vi "S4GUI.vi"(7 "Tab ObsEng":enum32{"Obs", "CCD modes", "Eng"}(tab)) -> ()   [LabVIEW 2018]
uses:
  S4GUI/S4GUI.lvclass
  S4GUI/S4GUI.lvclass/S4GUI.ctl
  Interface/Interface.lvclass/Interface.ctl
  Channel/Channel.lvclass/Channel.ctl
  Instrument/Instrument.lvclass/Instrument.ctl
  Device/Optics/Optics.lvclass/Optics.ctl
  Server/Server.lvclass/Server.ctl
  Device/Optics/Opt_Selector/Opt_Selector.lvclass
  C:/Users/devstaff/sparc4/s4gui/Versao ZeroMQ REQ-REP/SPARC4_GUI -20241112/Device/Optics/Optics.lvclass
  Device/Optics/Opt_Continuous/Opt_Continuous.lvclass
  SyncBox/Sync Box.lvclass
  C:/Users/devstaff/sparc4/s4gui/Versao ZeroMQ REQ-REP/SPARC4_GUI -20241112/Server/Server.lvclass
  Acquisition/Acquisition.lvclass
  Instrument/Instrument.lvclass
  Channel/Channel.lvclass
  TelFocus/TelFocus.lvclass
  Interface/Interface.lvclass
  StateMachine/State Machine.lvclass
  TCS/TCS.lvclass
  Publisher/Publisher.lvclass
  Trigger/Trigger.lvclass
  SecMirror/SecMirror.lvclass
  Device/Optics/Optics.lvclass
  Server/Server.lvclass
  Comm/Stream/Stream.lvclass
panel:
  out "GUI version":string
  out "LedExtSync":bool
  out "Name":string
  out "Angle":string
  out "Last Error":string
  in  "Tab Control 3":enum32{"Page 1"}(tab)
  in  "set Observer":bool
  out "Weather":bool
  out "Focus 160":bool
  in  "Observer":string
  out "S4ICSoft":bool
  out "Sync Box":bool
  out "Channel 4":bool
  out "Channel 3":bool
  out "Channel 2":bool
  out "Channel 1":bool
  out "GUIDER":bool
  out "TCSPD":bool
  in  "exit":bool
  out "RA":string
  out "DEC":string
  out "Julian Date":string
  out "Hour Angle":string
  out "Sideral Time":string
  out "Air Mass":string
  out "Date":string
  out "Telescope Focus":string
  out "Outside Temp":string
  out "Wind Speed[Km/h]":string
  out "Pressure":string
  out "Humidity":string
  in  "Project ID":string
  out "error out 8":errorcluster
  out "error out 7":errorcluster
  out "Readout\nRate":u8
  out "error out 6":errorcluster
  out "error out 5":errorcluster
  out "error out 4":errorcluster
  out "error out 3":errorcluster caption="error out"
  out "error out 2":errorcluster caption="error out"
  in  "S4ACS_GUI.lvclass":refnum<class "S4GUI.lvclass">
  out "Panel cooler 4":bool caption="Cooler"
  in  "set keywords":bool
  out "setupCH4":bool caption="Boolean"
  in  "Start ch4":bool
  in  "Pause ch4":bool
  in  "Stop ch4":bool
  in  "Abort ch4":bool
  out "Acq status string ch4":string
  out "setupCH3":bool caption="Boolean"
  in  "Start ch3":bool
  in  "Pause ch3":bool
  in  "Stop ch3":bool
  in  "Abort ch3":bool
  out "Acq status string ch3":string
  out "setupCH1":bool caption="Boolean"
  in  "Pause ch1":bool
  in  "Abort ch1":bool
  in  "Stop ch1":bool
  in  "Start ch1":bool
  out "Acq status string ch1":string
  out "setupCH2":bool caption="Boolean"
  in  "Start ch2":bool
  in  "Pause ch2":bool
  in  "Stop ch2":bool
  in  "Abort ch2":bool
  out "Acq status string ch2":string
  out "RO4":string caption="Read"
  out "G4":string caption="Gain"
  out "B4":string caption="Binn"
  out "PA4":string caption="Pre Amp"
  out "EA4":string caption="Mode"
  out "SI4":string caption="Sub image"
  out "Panel Temp 4":i16 caption="current"
  out "FT4":bool caption="FT"
  out "RO3":string caption="Read"
  out "G3":string caption="Gain"
  out "B3":string caption="Binn"
  out "PA3":string caption="Pre Amp"
  out "EA3":string caption="Mode"
  out "SI3":string caption="Sub image"
  out "Panel cooler 3":bool caption="Cooler"
  out "Panel Temp 3":i16 caption="current"
  out "FT3":bool caption="FT"
  out "RO2":string caption="Read"
  out "G2":string caption="Gain"
  out "B2":string caption="Binn"
  out "PA2":string caption="Pre Amp"
  out "EA2":string caption="Mode"
  out "SI2":string caption="Sub Image"
  out "Panel cooler 2":bool caption="Cooler"
  out "Panel Temp 2":i16 caption="current"
  out "FT2":bool caption="FT"
  out "G1":string caption="Gain"
  out "B1":string caption="Binn"
  out "PA1":string caption="PreAmp"
  out "EA1":string caption="Mode"
  out "SI1":string caption="Sub Image"
  out "FT1":bool caption="FT"
  in  "Tab CH3":enum32{"Acquisition", "CCD temp"}(tab)
  out "Cycles Done ch3":u32(slide) caption="#Cycles Done 1" scale=0.0..1.0
  out "Exposures Done ch3":i32(slide) caption="#Exposures Done 1" scale=0.0..1.0
  in  "#cycles ch3":u32=1 caption="#cycles" min=1 step=1
  in  "Exptime ch3":dbl=1.0 min=1e-05 step=1e-05
  in  "Exp ch3":u32=1 min=1 step=1
  out "Exposure Time ch3":dbl(slide) caption="Exposure Time 0.10" scale=0.0..0.1
  out "Last Image ch3":string caption="Last Image"
  out "Disk Storage ch3":u16(slide) caption="Disk Storage 75%" scale=0.0..100.0
  in  "Ready to OFF 3":bool caption="Ready to Power Off"
  out "Ext Cooling  status 3":bool caption="Ext Cool"
  out "Liquid Type 3":string caption="Liquid Type"
  out "Temp Status 3":string caption="Temp Status"
  out "Curr Temp 3":i16=1 min=1 step=1
  in  "Set Temp 3":bool
  in  "Target Temp 3":i32=1 caption="Target (C)" max=30
  out "Cooler status 3":bool caption="Cooler status"
  in  "Cooler 3":bool caption="Cooler"
  in  "Tab CH1":enum32{"Acquisition", "CCD temp"}(tab)
  out "Exposures Done ch1":i32(slide) caption="#Exposures Done 1" scale=0.0..1.0
  in  "Exptime ch1":dbl=1.0 min=1e-05 step=1e-05 format="%#.6g"
  in  "Exp ch1":u32=1 min=1 step=1
  out "Exposure Time ch1":dbl(slide) caption="Exposure Time 0.10" scale=0.0..0.1
  out "Last Image ch1":string caption="Last Image"
  out "Disk Storage ch1":u16(slide) caption="Disk Storage 52%" scale=0.0..100.0
  out "Cycles Done ch1":u32(slide) caption="#Cycles Done 1" scale=0.0..1.0
  in  "#cycles ch1":u32=1 caption="#cycles" min=1 step=1
  in  "Ready to OFF":bool caption="Ready to Power Off"
  out "Ext Cooling  status 1":bool caption="Ext Cool"
  out "Liquid Type 1":string caption="Liquid Type"
  in  "Set Temp 1":bool
  out "Temp Status 1":string caption="Temp Status"
  out "Cooler status 1":bool caption="Cooler status"
  in  "Target Temp 1":i8=1 caption="Target (C)" max=30
  in  "Cooler 1":bool caption="Cooler"
  out "Curr Temp 1":i16=1 min=1 step=1
  in  "Tab CH4":enum32{"Acquisition", "CCD temp"}(tab)
  out "Cycles Done ch4":u32(slide) caption="#Cycles Done 1" scale=0.0..1.0
  out "Exposures Done ch4":i32(slide) caption="#Exposures Done 1" scale=0.0..1.0
  in  "Exptime ch4":dbl=1.0 min=1e-05 step=1e-05
  in  "Exp ch4":u32=1 min=1 step=1
  in  "#cycles ch4":u32=1 caption="#cycles" min=1 step=1
  out "Exposure Time ch4":dbl(slide) caption="Exposure Time 0.10" scale=0.0..0.1
  out "Last Image ch4":string caption="Last Image"
  out "Disk Storage ch4":u16(slide) caption="Disk Storage 59%" scale=0.0..100.0
  in  "Ready to OFF 4":bool caption="Ready to Power Off"
  out "Ext Cooling  status 4":bool caption="Ext Cool"
  out "Liquid Type 4":string caption="Liquid Type"
  out "Temp Status 4":string caption="Temp Status"
  out "Curr Temp 4":i16=1 min=1 step=1
  in  "Set Temp 4":bool
  in  "Target Temp 4":i32=1 caption="Target (C)" max=30
  out "Cooler status 4":bool caption="Cooler status"
  in  "Cooler 4":bool caption="Cooler"
  in  "Pause SM":bool
  in  "Set Waveplate":bool
  in  "Calibrator Selector":u16(ring) items=["OFF", "POLARIZER", "PINHOLE", "SHUTTER", "DEPOLARIZER"]
  in  "Lambda Selector":u16(ring) items=["OFF", "Lambda/2", "Lambda/4"]
  in  "Select Positions":u16(ring) items=["All 16 positions", "First 8 positions", "First 4 positions", "1-4 & 9-12", "Clear", "Customized"]
  in  "P15":bool
  in  "P14":bool
  in  "P13":bool
  in  "P12":bool
  in  "P11":bool
  in  "P10":bool
  in  "P9":bool
  in  "P8":bool
  in  "P7":bool
  in  "P6":bool
  in  "P5":bool
  in  "P4":bool
  in  "P3":bool
  in  "P2":bool
  in  "P1":bool
  in  "P0":bool caption="1"
  out "Polarimetric Mode":bool
  out "Waveplate":bool
  out "WaveplatePos 2":dbl
  out "ledP0":bool
  out "ledP1":bool
  out "ledP2":bool
  out "ledP3":bool
  out "ledP4":bool
  out "ledP5":bool
  out "ledP6":bool
  out "ledP7":bool
  out "ledP8":bool
  out "ledP9":bool
  out "ledP10":bool
  out "ledP11":bool
  out "ledP12":bool
  out "ledP13":bool
  out "ledP14":bool
  out "ledP15":bool
  out "#Pol. Seq. Done":u32(slide) caption="#Pol. Seq. Done 0" scale=0.0..1.0
  out "#Cycles Done":u32(slide) caption="#Cycles Done 0" scale=0.0..1.0
  in  "Set SM":bool
  in  "SSM":u16(ring) items=["Asynchronous", "Synchronous by Cycle"]
  out "On SM":bool
  in  "# Cycles":u32=1 min=1 step=1
  in  "Abort SM":bool
  in  "Stop SM":bool
  in  "Start SM":bool
  in  "Index ch2":u32
  in  "Index ch3":u32
  in  "Index ch4":u32
  in  "Fire manual":bool
  out "PCS":bool caption="Calibrator"
  out "Analyzer":bool
  out "Photometric Mode":bool caption="Photometric"
  in  "Tab CH2":enum32{"Acquisition", "CCD temp"}(tab)
  in  "#cycles ch2":u32=1 caption="#cycles" min=1 step=1
  in  "Exptime ch2":dbl=1.0 min=1e-05 step=1e-05
  in  "Exp ch2":u32=1 min=1 step=1
  out "Exposure Time ch2":dbl(slide) caption="Exposure Time 0.10" scale=0.0..0.1
  out "Exposures Done ch2":i32(slide) caption="#Exposures Done 1" scale=0.0..1.0
  out "Last Image ch2":string caption="Last Image"
  out "Disk Storage ch2":u16(slide) caption="Disk Storage 69%" scale=0.0..100.0
  out "Cycles Done ch2":u32(slide) caption="#Cycles Done 1" scale=0.0..1.0
  in  "Ready to OFF 2":bool caption="Ready to Power Off"
  out "Ext Cooling  status 2":bool caption="Ext Cool"
  out "Liquid Type 2":string caption="Liquid Type"
  out "Temp Status 2":string caption="Temp Status"
  out "Curr Temp 2":i16=1 min=1 step=1
  in  "Set Temp 2":bool
  in  "Target Temp 2":i32=1 caption="Target (C)" max=30
  out "Cooler status 2":bool caption="Cooler status"
  in  "Cooler 2":bool caption="Cooler"
  in  "Tab Acq Type":T1(tab)
  in  "object suffix":string caption="filename suffix"
  in  "OBJECT Comments":string caption="Comments"
  in  "Object_obj":string caption="Object"
  in  "dflat suffix":string="DFLAT" caption="filename suffix"
  in  "DFLAT Comments":string caption="Comments"
  in  "Object_dflat":string="DOMEFLAT" caption="Object"
  in  "sflat suffix":string="SFLAT" caption="filename suffix"
  in  "SFLAT Comments":string caption="Comments"
  in  "Object_sflat":string="SKY FLAT" caption="Object"
  in  "dark suffix":string="DARK" caption="filename suffix"
  in  "DARK Comments":string caption="Comments"
  in  "Object_dark":string caption="Object"
  in  "ZERO Comments":string caption="Comments"
  in  "Object_zero":string="ZERO" caption="Object"
  in  "zero suffix":string="ZERO" caption="filename suffix"
  out "steps done":u32=1 caption="Step" min=1 step=1
  in  "#steps":u32=1 min=1 step=1
  in  "Step focus":i32=1 caption="Step" min=1 step=1
  in  "Start focus":i32=1 caption="Start" min=1 step=1
  in  "focus suffix":string="FOCUS" caption="filename suffix"
  in  "FOCUS Comments":string caption="Comments"
  in  "Object_focus":string caption="Object"
  in  "Stop Focus 2":bool
  in  "Set Focus 2":bool
  in  "Target focus 2":i32=1 caption="Target" min=1 step=1
  out "Target Temp 1":string caption="target"
  out "RO1":string caption="Read"
  out "Panel cooler 1":bool caption="Cooler"
  out "Panel Temp":i16 caption="current"
  out "Target Temp 2":string caption="target"
  out "Target Temp 3":string caption="target"
  out "Target Temp 4":string caption="target"
  out "SET CCD status":bool
  out "SET Temp status":bool
  out "Preview Temp.":dbl
  in  "enter password 2":bool caption="enter password"
  in  "password 2":string caption="password:"
  in  "EM Gain":u16=2 min=2 max=300 step=1
  out "InfoCCDmode":T2 caption="INFORMATION OF SELECTED MODE"
  in  "SZM":T3(ring) caption="Size mode"
  in  "AQM":T4(ring) caption="Acquisition Mode"
  in  "FTM":enum16{"OFF", "ON"}(ring) caption="Frame Transfer"
  in  "Set CCD mode":bool
  out "Parameters CCD modes":T5={"Image \nInitial Line"=0, "Image\nInitial Column"=0, "Image\nFinal Line"=0, "Image\nFInal Column"=0, "Vertical\nBinning"=0, "Horizontal\nBinning"=0, "Pre-amplification\nGain"=0, "CCD\nEM Gain"=2, "Readout\nRate"=0, "Shutter\nOpenning Time"=1, "Shutter\nClosing Time"=1, "Vertical\nShift Speed"=0, "Read\nMode"=0, "Vertical\nClock Voltage"=0, "A/D \nChannel"=0, "Shutter\nMode"=0, "Shutter\nTTL"=0, "Trigger\nMode"=0, "Frame\nTransfer"=FALSE, "Acquisition\nMode"=0, "CCD \nEM Mode"=0} caption="Preview Configuration for all channels:" {"CCD \nEM Mode" items=["Electron Mult.", "Conventional"]; "Acquisition\nMode" items=["None", "Single Scan", "Accumulate", "Kinectics", "Fast Kinectics", "None2", "Frame Transfer", "None3", "None4", "Time Delayed Integration"]; "Trigger\nMode" items=["Internal"=0, "Ext. Start"=6]; "Shutter\nTTL" items=["High", "Low"]; "Shutter\nMode" items=["Open"=1, "Closed"=2]; "Vertical\nClock Voltage" items=["Normal", "+1", "+2", "+3", "+4"]; "Read\nMode" items=["Full-Vertical-Binning", "Multi-Track", "Random-Track", "Single-Track", "Image"]; "Vertical\nShift Speed" items=["0.6", "1.13", "2.2", "4.33"]; "Shutter\nClosing Time" min=1; "Shutter\nOpenning Time" min=1; "Readout\nRate" items=["1 MHz", "0.1 MHz"]; "CCD\nEM Gain" min=2 max=300 step=1; "Pre-amplification\nGain" items=["Gain 1", "Gain 2"]}
  in  "Tab setup":T6(tab)
  out "Cameras Cluster":T7={"Current Configuration"={"Image Initial Line"=1.0, "Image Initial Column"=1.0, "Image Final Line"=1024.0, "Image FInal Column"=1024.0, "Vertical Binning"=1.0, "Horizontal Binning"=1.0, "Pre-amplification Gain"=0, "CCD EM Gain"=2, "Readout Rate"=0, "Shutter Openning Time"=50, "Shutter Closing Time"=50, "Vertical Shift Speed"=3, "Read Mode"=4, "Vertical Clock Voltage"=0, "A/D  Channel"=0, "Image Initial Line 2"=1.0, "Image Initial Column 2"=1.0, "Image Final Line 2"=1024.0, "Image FInal Column 2"=1024.0, "Vertical Binning 2"=1.0, "Horizontal Binning 2"=1.0, "Pre-amplification Gain 2"=0, "CCD EM Gain 2"=2, "Readout Rate 2"=0, "Shutter Openning Time 2"=50, "Shutter Closing Time 2"=50, "Vertical Shift Speed 2"=3, "Read Mode 2"=4, "Vertical Clock Voltage 2"=0, "A/D Channel 2"=0, "Image Initial Line 3"=1.0, "Image Initial Column 3"=1.0, "Image Final Line 3"=1024.0, "Image FInal Column 3"=1024.0, "Vertical Binning 3"=1.0, "Horizontal Binning 3"=1.0, "Pre-amplification Gain 3"=0, "CCD EM Gain 3"=2, "Readout Rate 3"=0, "Shutter Openning Time 3"=50, "Shutter Closing Time 3"=50, "Vertical Shift Speed 3"=3, "Read Mode 3"=4, "Vertical Clock Voltage 3"=0, "A/D Channel 3"=0, "Image Initial Line 4"=1.0, "Image Initial Column 4"=1.0, "Image Final Line 4"=1024.0, "Image FInal Column 4"=1024.0, "Vertical Binning 4"=1.0, "Horizontal Binning 4"=1.0, "Pre-amplification Gain 4"=0, "CCD EM Gain 4"=2, "Readout Rate 4"=0, "Shutter Openning Time 4"=50, "Shutter Closing Time 4"=50, "Vertical Shift Speed 4"=3, "Read Mode 4"=4, "Vertical Clock Voltage 4"=0, "A/D Channel 4"=0, "CCD EM Mode 2"=1, "CCD EM Mode 3"=1, "CCD EM Mode 4"=1, "CCD EM Mode"=1, "Shutter Mode"=2, "Shutter Mode 2"=2, "Shutter Mode 4"=2, "Shutter Mode 3"=2, "Shutter TTL"=1, "Shutter TTL 2"=1, "Shutter TTL 3"=1, "Shutter TTL 4"=1, "Frame Transfer"=TRUE, "Frame Transfer 2"=TRUE, "Frame Transfer 3"=TRUE, "Frame Transfer 4"=TRUE, "Trigger Mode"=0, "Trigger Mode 2"=0, "Trigger Mode 3"=0, "Trigger Mode 4"=0, "Acquisition Mode"=3, "Acquisition Mode 2"=3, "Acquisition Mode 3"=3, "Acquisition Mode 4"=3}} {"Current Configuration"."Acquisition Mode 4" items=["", "Single Scan", "Accumulate", "Kinectics", "Fast Kinectics", "None2", "Frame Transfer", "None3", "None4", "Time Delayed Integration"]; "Current Configuration"."Acquisition Mode 3" items=["None", "Single Scan", "Accumulate", "Kinectics", "Fast Kinectics", "None2", "Frame Transfer", "None3", "None4", "Time Delayed Integration"]; "Current Configuration"."Acquisition Mode 2" items=["None", "Single Scan", "Accumulate", "Kinectics", "Fast Kinectics", "None2", "Frame Transfer", "None3", "None4", "Time Delayed Integration"]; "Current Configuration"."Acquisition Mode" items=["None", "Single Scan", "Accumulate", "Kinectics", "Fast Kinectics", "None2", "Frame Transfer", "None3", "None4", "Time Delayed Integration"]; "Current Configuration"."Trigger Mode 4" items=["Internal"=0, "Ext. Start"=6]; "Current Configuration"."Trigger Mode 3" items=["Internal"=0, "Ext. Start"=6]; "Current Configuration"."Trigger Mode 2" items=["Internal"=0, "Ext. Start"=6]; "Current Configuration"."Trigger Mode" items=["Internal"=0, "Ext. Start"=6]; "Current Configuration"."Shutter TTL 4" items=["High", "Low"]; "Current Configuration"."Shutter TTL 3" items=["High", "Low"]; "Current Configuration"."Shutter TTL 2" items=["High", "Low"]; "Current Configuration"."Shutter TTL" items=["High", "Low"]; "Current Configuration"."Shutter Mode 3" items=["Open"=1, "Closed"=2]; "Current Configuration"."Shutter Mode 4" items=["Open"=1, "Closed"=2]; "Current Configuration"."Shutter Mode 2" items=["Open"=1, "Closed"=2]; "Current Configuration"."Shutter Mode" items=["Open"=1, "Closed"=2]; "Current Configuration"."CCD EM Mode" items=["Electron Mult.", "Conventional"]; "Current Configuration"."CCD EM Mode 4" items=["Electron Mult.", "Conventional"]; "Current Configuration"."CCD EM Mode 3" items=["Electron Mult.", "Conventional"]; "Current Configuration"."CCD EM Mode 2" items=["Electron Mult.", "Conventional"]; "Current Configuration"."Vertical Clock Voltage 4" items=["Normal", "+1", "+2", "+3", "+4"]; "Current Configuration"."Read Mode 4" items=["Full-Vertical-Binning", "Multi-Track", "Random-Track", "Single-Track", "Image"]; "Current Configuration"."Vertical Shift Speed 4" items=["0.6", "1.13", "2.2", "4.33"]; "Current Configuration"."Readout Rate 4" items=["1 MHz", "0.1 MHz"]; "Current Configuration"."Pre-amplification Gain 4" items=["Gain 1", "Gain 2"]; "Current Configuration"."Vertical Clock Voltage 3" items=["Normal", "+1", "+2", "+3", "+4"]; "Current Configuration"."Read Mode 3" items=["Full-Vertical-Binning", "Multi-Track", "Random-Track", "Single-Track", "Image"]; "Current Configuration"."Vertical Shift Speed 3" items=["0.6", "1.13", "2.2", "4.33"]; "Current Configuration"."Readout Rate 3" items=["1 MHz", "0.1 MHz"]; "Current Configuration"."Pre-amplification Gain 3" items=["Gain 1", "Gain 2"]; "Current Configuration"."Vertical Clock Voltage 2" items=["Normal", "+1", "+2", "+3", "+4"]; "Current Configuration"."Read Mode 2" items=["Full-Vertical-Binning", "Multi-Track", "Random-Track", "Single-Track", "Image"]; "Current Configuration"."Vertical Shift Speed 2" items=["0.6", "1.13", "2.2", "4.33"]; "Current Configuration"."Readout Rate 2" items=["1 MHz", "0.1 MHz"]; "Current Configuration"."Pre-amplification Gain 2" items=["Gain 1", "Gain 2"]; "Current Configuration"."Vertical Clock Voltage" items=["Normal", "+1", "+2", "+3", "+4"]; "Current Configuration"."Read Mode" items=["Full-Vertical-Binning", "Multi-Track", "Random-Track", "Single-Track", "Image"]; "Current Configuration"."Vertical Shift Speed" items=["0.6", "1.13", "2.2", "4.33"]; "Current Configuration"."Readout Rate" items=["1 MHz", "0.1 MHz"]; "Current Configuration"."Pre-amplification Gain" items=["Gain 1", "Gain 2"]}
  in  "Input Cluster":T8={"Parameters"={"Image \nInitial Line"=0, "Image\nInitial Column"=0, "Image\nFinal Line"=0, "Image\nFInal Column"=0, "Vertical\nBinning"=0, "Horizontal\nBinning"=0, "Pre-amplification\nGain"=0, "CCD\nEM Gain"=2, "Readout\nRate"=0, "Shutter\nOpenning Time"=1, "Shutter\nClosing Time"=1, "Vertical\nShift Speed"=0, "Read\nMode"=0, "Vertical\nClock Voltage"=0, "A/D \nChannel"=0, "Shutter\nMode"=0, "Shutter\nTTL"=0, "Trigger\nMode"=0, "Frame\nTransfer"=FALSE, "Acquisition\nMode"=0, "CCD \nEM Mode"=0}} {"Parameters"."CCD \nEM Mode" items=["Electron Mult.", "Conventional"]; "Parameters"."Acquisition\nMode" items=["None", "Single Scan", "Accumulate", "Kinectics", "Fast Kinectics", "None2", "Frame Transfer", "None3", "None4", "Time Delayed Integration"]; "Parameters"."Trigger\nMode" items=["Internal"=0, "Ext. Start"=6]; "Parameters"."Shutter\nTTL" items=["High", "Low"]; "Parameters"."Shutter\nMode" items=["Open"=1, "Closed"=2]; "Parameters"."Vertical\nClock Voltage" items=["Normal", "+1", "+2", "+3", "+4"]; "Parameters"."Read\nMode" items=["Full-Vertical-Binning", "Multi-Track", "Random-Track", "Single-Track", "Image"]; "Parameters"."Vertical\nShift Speed" items=["0.6", "1.13", "2.2", "4.33"]; "Parameters"."Shutter\nClosing Time" min=1; "Parameters"."Shutter\nOpenning Time" min=1; "Parameters"."Readout\nRate" items=["1 MHz", "0.1 MHz"]; "Parameters"."CCD\nEM Gain" min=2 max=300 step=1; "Parameters"."Pre-amplification\nGain" items=["Gain 1", "Gain 2"]}
  in  "enter password":bool
  in  "password":string caption="password:"
  in  "CH4 on":bool
  in  "CH3 on":bool
  in  "CH2on":bool
  in  "CH1on":bool
  out "CCD checked 4":bool
  out "CCD checked 3":bool
  out "CCD checked 2":bool
  out "CCD checked 1":bool
  in  "Load Default Button":bool
  in  "Save As Button":bool caption="Save"
  in  "Load Button":bool
  in  "Set from Input ch3":bool
  in  "Restore Default ch4":bool
  in  "Copy to Input ch4":bool
  in  "Set from Input ch4":bool
  in  "Restore Default ch3":bool
  in  "Copy to Input ch3":bool
  in  "Restore Default ch2":bool
  in  "Copy to Input ch2":bool
  in  "Set from Input ch2":bool
  in  "Restore Default ch1":bool
  in  "Copy to Input ch1":bool
  in  "Set from Input ch1":bool
  out "Current Configuration File:":string
  in  "Scrollbar":i32(c297)
  in  "Save Button":bool
  in  "Close Button":bool
  out "selected path":path
  out "loop max(ms)":u32
  out "loop time(ms)":u32
  in  "reset max":bool
  out "Status":string
  out "PosName ASEL":string
  out "PosName CALW":string
  out "GFOC Status":bool
  out "GMIR Status":bool
  out "ASEL Status":bool
  out "CALW Status":bool
  out "WPROT Status":bool
  out "WPSEL Status":bool
  in  "AllConfig":bool
  in  "TARGET NAME ASEL":enum16{"NONE", "OFF", "ON"}(ring) caption="TARGET NAME"
  in  "TARGET NAME CALW":T9(ring) caption="TARGET NAME"
  in  "TARGET NAME WPSEL":enum16{"NONE", "OFF", "L/2", "L/4"}(ring) caption="TARGET NAME"
  in  "TARGET NAME WPROT":T10(ring) caption="TARGET NAME"
  in  "ASEL_init":bool
  in  "CALW_init":bool
  in  "GFOC_init":bool
  in  "GMIR_init":bool
  in  "WPSEL_init":bool
  in  "WPROT_init":bool
  out "PosName ASEL":dbl
  out "Position CALW":dbl
  out "Position GFOC":dbl
  out "Position GMIR":dbl
  out "Position WPSEL":dbl
  out "Position WPROT":dbl
  in  "ASEL_stop":bool
  in  "ASEL_set":bool
  in  "ASEL_target":dbl caption="TARGET"
  in  "CALW_stop":bool
  in  "CALW_set":bool
  in  "CALW_target":dbl caption="TARGET"
  in  "GFOC_stop":bool
  in  "GFOC_set":bool
  in  "GFOC_target":dbl caption="TARGET"
  in  "GMIR_stop":bool
  in  "GMIR_set":bool
  in  "GMIR_target":dbl caption="TARGET"
  in  "WPSEL_stop":bool
  in  "WPSEL_set":bool
  in  "WPSEL_target":dbl caption="TARGET"
  in  "WPROT_stop":bool
  in  "WPROT_set":bool
  out "PosName WPSEL":string
  out "PosName WPROT":string
  in  "Init mode":bool caption="Initiating..."
  out "Current State":i32
  in  "SyncBox":bool
  in  "DelayD":string
  in  "DelayC":string
  in  "DelayB":string
  in  "DelayA":string
  in  "Set SyncBox":bool
  in  "WidthA":string
  in  "WidthB":string
  in  "WidthC":string
  in  "WidthD":string
  in  "Avança Estado":bool
  in  "Select Trigger Mode":bool
  out "String":string
  in  "Fire":bool
  out "String 2":string
  in  "Stop Focus":bool
  in  "Set Focus":bool
  in  "Target focus":i32=1 caption="Target" min=1 step=1
  in  "S4ICS protocol":bool
  out "Cycles Counter":i32
  in  "TCS mode":bool
  in  "Filter4":u8(ring) items=["CLEAR", "U", "B", "V", "R", "I"]
  in  "Filter3":u8(ring) items=["CLEAR", "U", "B", "V", "R", "I"]
  in  "Filter2":u8(ring) items=["CLEAR", "U", "B", "V", "R", "I"]
  in  "Filter1":u8(ring) items=["CLEAR", "U", "B", "V", "R", "I"]
  in  "Night Directory":string="C:\\Users\\observer\\Desktop\\SPARC4 Acquisition Control\\Imagens"
  out "DS9 2":bool
  in  "Channel DS9 Selector":u16(ring) items=["Channel 1", "Channel 2", "Channel 3", "Channel 4"]
  in  "Set Channel DS9":bool
  out "Channel 5":i32
  out "Channel 6":i32
  out "Channel 7":i32
  out "Channel 2a":i32
  out "Channel 3a":i32
  out "Channel 4a":i32
  in  "Run WPROT":bool caption="Run"
  in  "Ciclos  WPROT":u32 caption="Ciclos"
  in  "SendExpose":bool caption="SEND EXPOSE\n      COMM"
  out "error out 9":errorcluster
  out "error out":errorcluster
  out "All Pubs":T11
  # "SPARC4"
  # "Triggering Mode"
  # "Select Triggering Mode"
  # "Function Setup"
  # "TEMP"
  # "TEMP"
  # "TEMP"
  # "TEMP"
  # "Channel 4"
  # "Detector status"
  # "Channel 3"
  # "Detector status"
  # "Channel 1"
  # "Detector status"
  # "Channel 2"
  # "Detector status"
  # "ExpTime(s)"
  # "#Exp"
  # "#Cycles"
  # "(C)"
  # "ExpTime(s)"
  # "#Exp"
  # "#Cycles"
  # "(C)"
  # "ExpTime(s)"
  # "#Exp"
  # "#Cycles"
  # "(C)"
  # "Waveplate Selector"
  # "Polarimetric \nCalibrator Selector"
  # "Waveplate Sequence"
  # "1           4               8               12             16"
  # "ExpTime(s)"
  # "#Exp"
  # "#Cycles"
  # "(C)"
  # "If possible, use an OBJECT ID resolved by Simbad."
  # "Use the same OBJECT ID from OBJECT tab."
  # "Channel 1            Channel 2          Channel 3          Channel 4"
  # "ON"
  # "ON"
  # "ON"
  # "ON"
  # "Parameter Input"
  # "Current Configuration Parameters"
  # "Input to Channel:"
  # "Single channel \noperations:"
  # "Channel to Input:"
  # "Default to Channel:"
  # "File Operations:\n(apply for all channels)"
  # "Instrument"
  # "WPSEL"
  # "WPROT"
  # "CALW"
  # "ASEL"
  # "GMIR"
  # "GFOC"
  # "Select Trigger Mode"
  # "Extern"
  # "Remote"
  # "Telesc. focus"
  # "Teste S4ICS"
  # "Real"
  # "0MQ"
  # "Simul"
  # "TCP-IP"
  # "Number of exposures in the queue"
  # "Automatic DS9 Display"
  # "Enter observer's name"
  # "FILTER"
  # "channel 1"
  # "channel 2"
  # "channel 3"
  # "channel 4"
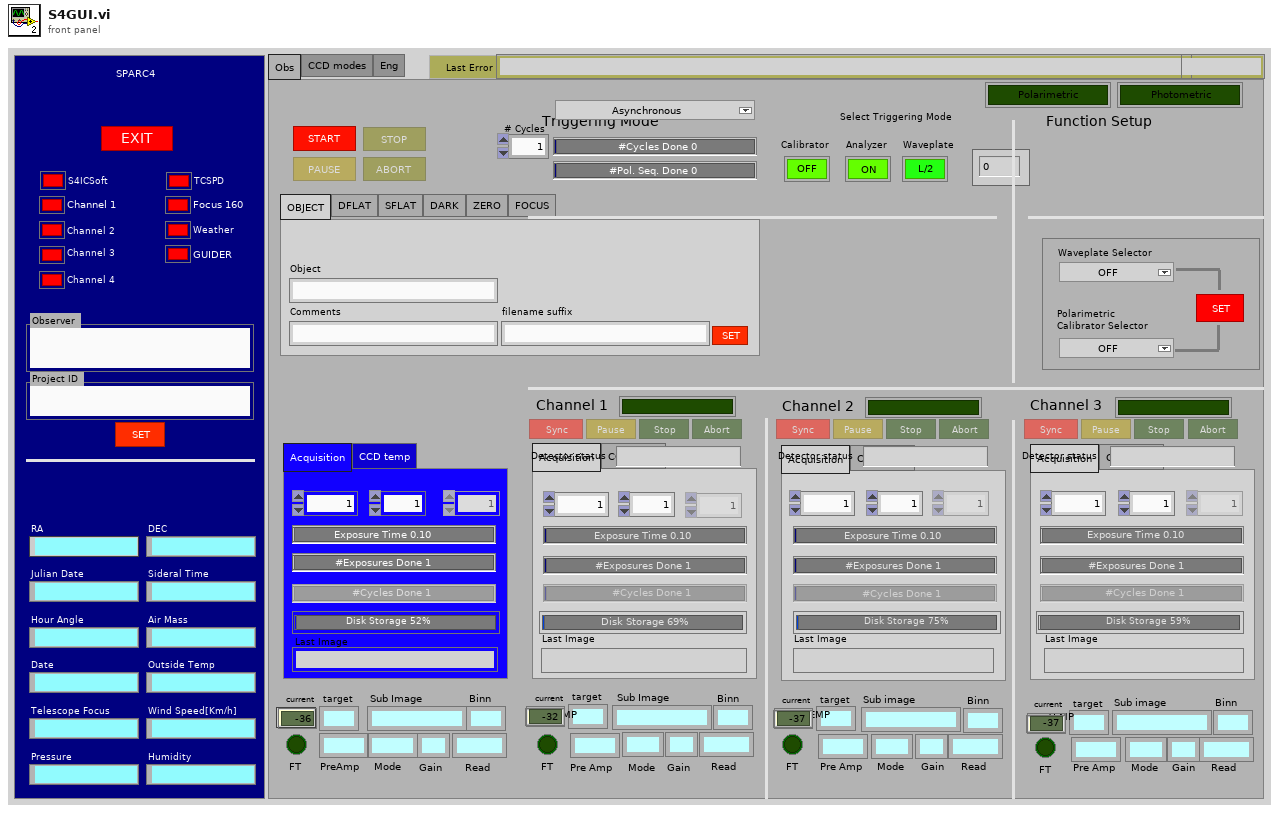
[diagram p1: front panel]
types:
  T1 = enum32{"OBJECT", "DFLAT", "SFLAT", "DARK", "ZERO", "FOCUS"}
  T2 = cluster{"AcqRate":dbl, "MinExpTime":dbl, "readNoise":dbl, "readTime":dbl, "SatLim":dbl}
  T3 = enum16{"LARGE: FoV=5.6' / Pix=0.3\"", "LARGE: FoV=5.6' / Pix=0.7\"", "MEDIUM: FoV=2.8'/ Pix=0.3\"", "MEDIUM: FoV=2.8' / Pix=0.7\"", "SMALL FoV=1.4' / Pix=0.3\"", "SMALL: FoV=1.4' / Pix=0.7\""}
  T4 = enum16{"SLOW BRIGHT: Conventional; 0.1 MHz; Gain 1", "SLOW FAINT: Conventional; 0.1 MHz; Gain 2", "NORMAL BRIGHT: Conventional; 1 MHz; Gain 1", "NORMAL FAINT: Conventional; 1 MHz; Gain 2", "FAST: EM; 10 MHz", "FAST+: EM; 20 MHz", "SUPERFAST: EM; 30 MHz"}
  T5 = cluster{"Image \nInitial Line":u16, "Image\nInitial Column":u16, "Image\nFinal Line":u16, "Image\nFInal Column":u16, "Vertical\nBinning":u16, "Horizontal\nBinning":u16, "Pre-amplification\nGain":u8, "CCD\nEM Gain":u16, "Readout\nRate":u8, "Shutter\nOpenning Time":i32, "Shutter\nClosing Time":i32, "Vertical\nShift Speed":u8, "Read\nMode":u8, "Vertical\nClock Voltage":u8, "A/D \nChannel":u32, "Shutter\nMode":u16, "Shutter\nTTL":u16, "Trigger\nMode":u16, "Frame\nTransfer":bool, "Acquisition\nMode":u8, "CCD \nEM Mode":u8}
  T6 = enum32{"Camera", "Instrument", "SyncBox", "Other Setup", "Pub info"}
  T7 = cluster{"Current Configuration":cluster{"Image Initial Line":dbl, "Image Initial Column":dbl, "Image Final Line":dbl, "Image FInal Column":dbl, "Vertical Binning":dbl, "Horizontal Binning":dbl, "Pre-amplification Gain":u8, "CCD EM Gain":u8, "Readout Rate":u8, "Shutter Openning Time":i32, "Shutter Closing Time":i32, "Vertical Shift Speed":u8, "Read Mode":u8, "Vertical Clock Voltage":u8, "A/D  Channel":u32, "Image Initial Line 2":dbl, "Image Initial Column 2":dbl, "Image Final Line 2":dbl, "Image FInal Column 2":dbl, "Vertical Binning 2":dbl, "Horizontal Binning 2":dbl, "Pre-amplification Gain 2":u8, "CCD EM Gain 2":u16, "Readout Rate 2":u8, "Shutter Openning Time 2":i32, "Shutter Closing Time 2":i32, "Vertical Shift Speed 2":u8, "Read Mode 2":u8, "Vertical Clock Voltage 2":u8, "A/D Channel 2":u32, "Image Initial Line 3":dbl, "Image Initial Column 3":dbl, "Image Final Line 3":dbl, "Image FInal Column 3":dbl, "Vertical Binning 3":dbl, "Horizontal Binning 3":dbl, "Pre-amplification Gain 3":u8, "CCD EM Gain 3":u16, "Readout Rate 3":u8, "Shutter Openning Time 3":i32, "Shutter Closing Time 3":i32, "Vertical Shift Speed 3":u8, "Read Mode 3":u8, "Vertical Clock Voltage 3":u8, "A/D Channel 3":u32, "Image Initial Line 4":dbl, "Image Initial Column 4":dbl, "Image Final Line 4":dbl, "Image FInal Column 4":dbl, "Vertical Binning 4":dbl, "Horizontal Binning 4":dbl, "Pre-amplification Gain 4":u8, "CCD EM Gain 4":u16, "Readout Rate 4":u8, "Shutter Openning Time 4":i32, "Shutter Closing Time 4":i32, "Vertical Shift Speed 4":u8, "Read Mode 4":u8, "Vertical Clock Voltage 4":u8, "A/D Channel 4":u32, "CCD EM Mode 2":u8, "CCD EM Mode 3":u8, "CCD EM Mode 4":u8, "CCD EM Mode":u16, "Shutter Mode":u16, "Shutter Mode 2":u16, "Shutter Mode 4":u16, "Shutter Mode 3":u16, "Shutter TTL":u16, "Shutter TTL 2":u16, "Shutter TTL 3":u16, "Shutter TTL 4":u16, "Frame Transfer":bool, "Frame Transfer 2":bool, "Frame Transfer 3":bool, "Frame Transfer 4":bool, "Trigger Mode":u16, "Trigger Mode 2":u16, "Trigger Mode 3":u16, "Trigger Mode 4":u16, "Acquisition Mode":u8, "Acquisition Mode 2":u8, "Acquisition Mode 3":u8, "Acquisition Mode 4":u8}}
  T8 = cluster{"Parameters":cluster{"Image \nInitial Line":u16, "Image\nInitial Column":u16, "Image\nFinal Line":u16, "Image\nFInal Column":u16, "Vertical\nBinning":u16, "Horizontal\nBinning":u16, "Pre-amplification\nGain":u8, "CCD\nEM Gain":u16, "Readout\nRate":u8, "Shutter\nOpenning Time":i32, "Shutter\nClosing Time":i32, "Vertical\nShift Speed":u8, "Read\nMode":u8, "Vertical\nClock Voltage":u8, "A/D \nChannel":u32, "Shutter\nMode":u16, "Shutter\nTTL":u16, "Trigger\nMode":u16, "Frame\nTransfer":bool, "Acquisition\nMode":u8, "CCD \nEM Mode":u8}}
  T9 = enum16{"NONE", "OFF", "POLARIZER", "PINHOLE", "SHUTTER", "DEPOLARIZER"}
  T10 = enum16{"NONE", "WP1", "WP2", "WP3", "WP4", "WP5", "WP6", "WP7", "WP8", "WP9", "WP10", "WP11", "WP12", "WP13", "WP14", "WP15", "WP16"}
  T11 = cluster{"PubACS1":string, "PubACS2":string, "PubACS3":string, "PubACS4":string, "PubICS":string, "PubTCS":string, "PubFocus160":string, "PubWeather":string, "PubGS":string, "PubS4GUI":string}
  T12 = enum8{"Enabled", "Disabled", "Disabled and Grayed Out"}
  T13 = cluster{"Parameters":refnum<vi>, "Current Configuration":refnum<vi>}
  T14 = cluster{"ACQUISITION_MODE":bool, "TRIGGER_MODE":bool, "READ_MODE":bool, "PREAMP":bool, "READOUT_RATE":bool, "VERTICAL_SHIFT_SPEED":bool, "EM_MODE":bool, "EM_GAIN":bool, "SHUTTER_MODE":bool, "SHUTTER_TTL":bool, "SHUTTER_OPENING_TIME":bool, "SHUTTER_CLOSING_TIME":bool, "VBIN":bool, "HBIN":bool, "INITIAL_LINE":bool, "INITIAL_COLUMN":bool, "FINAL_LINE":bool, "FINAL_COLUMN":bool, "FRAME_TRANSFER":bool, "VERTICAL_CLOCK_VOLTAGE":bool, "AD_CHANNEL":bool}
  T15 = cluster{"Trigger Mode Status":string, "String output":string, "Instrument Status":cluster{"WPROT pos":dbl, "WPSEL pos":dbl, "GMIR pos":dbl, "GFOC pos":dbl, "CALW pos":dbl, "ASEL pos":dbl, "mode":bool, "String Status":string, "connection":bool, "operational":bool}, "Sync Box State":i32, "Trigger General Status":string, "Instrument States":cluster{"WPSEL State":i32, "WPROT State":i32, "CALW State":i32, "ASEL State":i32, "GMIR State":i32, "GFOC State":i32}, "Instrument Pos Names":cluster{"WPROT posname":string, "WPSEL posname":string, "CALW posname":string, "ASEL posname":string}, "ChannelA_Status":cluster{"Current exp":dbl, "Frames done":u32, "LastFileImage":string, "CamStatus":string, "Run state":u32, "connection":bool, "Cooler ON/OFF":i16, "Currently temperature":i16, "Temperature Status":string, "target  temp":i16, "conf runing":bool, "FT":bool, "UsedDisk":u16, "operational":bool}, "WPROT seq":u16, "ChannelB_Status":cluster{"Current exp":dbl, "Frames done":u32, "LastFileImage":string, "CamStatus":string, "Run state":u32, "connection":bool, "Cooler ON/OFF":i16, "Currently temperature":i16, "Temperature Status":string, "target  temp":i16, "conf runing":bool, "FT":bool, "UsedDisk":u16, "operational":bool}, "ChannelC_Status":cluster{"Current exp":dbl, "Frames done":u32, "LastFileImage":string, "CamStatus":string, "Run state":u32, "connection":bool, "Cooler ON/OFF":i16, "Currently temperature":i16, "Temperature Status":string, "target  temp":i16, "conf runing":bool, "FT":bool, "UsedDisk":u16, "operational":bool}, "ChannelD_Status":cluster{"Current exp":dbl, "Frames done":u32, "LastFileImage":string, "CamStatus":string, "Run state":u32, "connection":bool, "Cooler ON/OFF":i16, "Currently temperature":i16, "Temperature Status":string, "target  temp":i16, "conf runing":bool, "FT":bool, "UsedDisk":u16, "operational":bool}, "ChannelA_CCD":cluster{"ACQUISITION_MODE":u8, "TRIGGER_MODE":u8, "READ_MODE":u8, "PREAMP":u8, "READOUT_RATE":u8, "VERTICAL_SHIFT_SPEED":u8, "EM_MODE":u8, "EM_GAIN":u16, "SHUTTER_MODE":u8, "SHUTTER_TTL":u8, "SHUTTER_OPENNING_TIME":u16, "SHUTTER_CLOSING_TIME":u16, "VBIN":u16, "HBIN":u16, "INITIAL_LINE":u16, "INITIAL_COLUMN":u16, "FINAL_LINE":u16, "FINAL_COLUMN":u16, "FRAME_TRANSFER":bool, "VERTICAL_CLOCK_VOLTAGE":u8, "AD_CHANNEL":u32}, "ChannelB_CCD ":cluster{"ACQUISITION_MODE":u8, "TRIGGER_MODE":u8, "READ_MODE":u8, "PREAMP":u8, "READOUT_RATE":u8, "VERTICAL_SHIFT_SPEED":u8, "EM_MODE":u8, "EM_GAIN":u16, "SHUTTER_MODE":u8, "SHUTTER_TTL":u8, "SHUTTER_OPENNING_TIME":u16, "SHUTTER_CLOSING_TIME":u16, "VBIN":u16, "HBIN":u16, "INITIAL_LINE":u16, "INITIAL_COLUMN":u16, "FINAL_LINE":u16, "FINAL_COLUMN":u16, "FRAME_TRANSFER":bool, "VERTICAL_CLOCK_VOLTAGE":u8, "AD_CHANNEL":u32}, "ChannelC_CCD":cluster{"ACQUISITION_MODE":u8, "TRIGGER_MODE":u8, "READ_MODE":u8, "PREAMP":u8, "READOUT_RATE":u8, "VERTICAL_SHIFT_SPEED":u8, "EM_MODE":u8, "EM_GAIN":u16, "SHUTTER_MODE":u8, "SHUTTER_TTL":u8, "SHUTTER_OPENNING_TIME":u16, "SHUTTER_CLOSING_TIME":u16, "VBIN":u16, "HBIN":u16, "INITIAL_LINE":u16, "INITIAL_COLUMN":u16, "FINAL_LINE":u16, "FINAL_COLUMN":u16, "FRAME_TRANSFER":bool, "VERTICAL_CLOCK_VOLTAGE":u8, "AD_CHANNEL":u32}, "ChannelD_CCD":cluster{"ACQUISITION_MODE":u8, "TRIGGER_MODE":u8, "READ_MODE":u8, "PREAMP":u8, "READOUT_RATE":u8, "VERTICAL_SHIFT_SPEED":u8, "EM_MODE":u8, "EM_GAIN":u16, "SHUTTER_MODE":u8, "SHUTTER_TTL":u8, "SHUTTER_OPENNING_TIME":u16, "SHUTTER_CLOSING_TIME":u16, "VBIN":u16, "HBIN":u16, "INITIAL_LINE":u16, "INITIAL_COLUMN":u16, "FINAL_LINE":u16, "FINAL_COLUMN":u16, "FRAME_TRANSFER":bool, "VERTICAL_CLOCK_VOLTAGE":u8, "AD_CHANNEL":u32}, "CHA_Checked Params":cluster{"ACQUISITION_MODE":bool, "TRIGGER_MODE":bool, "READ_MODE":bool, "PREAMP":bool, "READOUT_RATE":bool, "VERTICAL_SHIFT_SPEED":bool, "EM_MODE":bool, "EM_GAIN":bool, "SHUTTER_MODE":bool, "SHUTTER_TTL":bool, "SHUTTER_OPENING_TIME":bool, "SHUTTER_CLOSING_TIME":bool, "VBIN":bool, "HBIN":bool, "INITIAL_LINE":bool, "INITIAL_COLUMN":bool, "FINAL_LINE":bool, "FINAL_COLUMN":bool, "FRAME_TRANSFER":bool, "VERTICAL_CLOCK_VOLTAGE":bool, "AD_CHANNEL":bool}, "CHB_Checked Params":cluster{"ACQUISITION_MODE":bool, "TRIGGER_MODE":bool, "READ_MODE":bool, "PREAMP":bool, "READOUT_RATE":bool, "VERTICAL_SHIFT_SPEED":bool, "EM_MODE":bool, "EM_GAIN":bool, "SHUTTER_MODE":bool, "SHUTTER_TTL":bool, "SHUTTER_OPENING_TIME":bool, "SHUTTER_CLOSING_TIME":bool, "VBIN":bool, "HBIN":bool, "INITIAL_LINE":bool, "INITIAL_COLUMN":bool, "FINAL_LINE":bool, "FINAL_COLUMN":bool, "FRAME_TRANSFER":bool, "VERTICAL_CLOCK_VOLTAGE":bool, "AD_CHANNEL":bool}, "CHC_Checked Params":cluster{"ACQUISITION_MODE":bool, "TRIGGER_MODE":bool, "READ_MODE":bool, "PREAMP":bool, "READOUT_RATE":bool, "VERTICAL_SHIFT_SPEED":bool, "EM_MODE":bool, "EM_GAIN":bool, "SHUTTER_MODE":bool, "SHUTTER_TTL":bool, "SHUTTER_OPENING_TIME":bool, "SHUTTER_CLOSING_TIME":bool, "VBIN":bool, "HBIN":bool, "INITIAL_LINE":bool, "INITIAL_COLUMN":bool, "FINAL_LINE":bool, "FINAL_COLUMN":bool, "FRAME_TRANSFER":bool, "VERTICAL_CLOCK_VOLTAGE":bool, "AD_CHANNEL":bool}, "CHD_Checked Params":cluster{"ACQUISITION_MODE":bool, "TRIGGER_MODE":bool, "READ_MODE":bool, "PREAMP":bool, "READOUT_RATE":bool, "VERTICAL_SHIFT_SPEED":bool, "EM_MODE":bool, "EM_GAIN":bool, "SHUTTER_MODE":bool, "SHUTTER_TTL":bool, "SHUTTER_OPENING_TIME":bool, "SHUTTER_CLOSING_TIME":bool, "VBIN":bool, "HBIN":bool, "INITIAL_LINE":bool, "INITIAL_COLUMN":bool, "FINAL_LINE":bool, "FINAL_COLUMN":bool, "FRAME_TRANSFER":bool, "VERTICAL_CLOCK_VOLTAGE":bool, "AD_CHANNEL":bool}, "Trigger_connection":bool, "TCSPD_connection":bool, "TCS extended":string, "TCS id":u32, "S4ICS id":u32, "focus pos":i32, "Focus_connection":bool, "WS_connection":bool, "weather status":cluster{"broker":string, "version":string, "date":string, "hour":string, "outHumidity":string, "inHumidity":string, "inTemp":string, "outTemp":string, "windSpeed":string, "windDirection":string, "pressure":string, "dewOut":string, "dewIn":string, "leaf":string, "rain":string, "windChill":string}, "GS STATUS cluster":cluster{"FocusPhot":dbl, "FocusPolar":dbl, "FocusEffic":dbl, "FocusInstrum":dbl, "ICS":bool, "AG":bool, "BROKER":string}, "TCSPD_operational":bool, "Focus_operational":bool}
  T16 = cluster{"Cluster Mode Sync":cluster{"#Index Cycles":enum8{"Enabled", "Disabled", "Disabled and Grayed Out"}, "#Cycles":enum8{"Enabled", "Disabled", "Disabled and Grayed Out"}, "SSM":enum8{"Enabled", "Disabled", "Disabled and Grayed Out"}, "Set SM":enum8{"Enabled", "Disabled", "Disabled and Grayed Out"}, "Star SM":enum8{"Enabled", "Disabled", "Disabled and Grayed Out"}, "Pause SM":enum8{"Enabled", "Disabled", "Disabled and Grayed Out"}, "Stop SM":enum8{"Enabled", "Disabled", "Disabled and Grayed Out"}, "Abort SM":enum8{"Enabled", "Disabled", "Disabled and Grayed Out"}, "Start SM Text":string}, "Cluster Polarimetry":cluster{"Lambda Selector":enum8{"Enabled", "Disabled", "Disabled and Grayed Out"}, "Calibrator Selector":enum8{"Enabled", "Disabled", "Disabled and Grayed Out"}, "Set Waveplate":enum8{"Enabled", "Disabled", "Disabled and Grayed Out"}, "Select Positions":enum8{"Enabled", "Disabled", "Disabled and Grayed Out"}, "P0":enum8{"Enabled", "Disabled", "Disabled and Grayed Out"}, "P1":enum8{"Enabled", "Disabled", "Disabled and Grayed Out"}, "P2":enum8{"Enabled", "Disabled", "Disabled and Grayed Out"}, "P3":enum8{"Enabled", "Disabled", "Disabled and Grayed Out"}, "P4":enum8{"Enabled", "Disabled", "Disabled and Grayed Out"}, "P5":enum8{"Enabled", "Disabled", "Disabled and Grayed Out"}, "P6":enum8{"Enabled", "Disabled", "Disabled and Grayed Out"}, "P7":enum8{"Enabled", "Disabled", "Disabled and Grayed Out"}, "P8":enum8{"Enabled", "Disabled", "Disabled and Grayed Out"}, "P9":enum8{"Enabled", "Disabled", "Disabled and Grayed Out"}, "P10":enum8{"Enabled", "Disabled", "Disabled and Grayed Out"}, "P11":enum8{"Enabled", "Disabled", "Disabled and Grayed Out"}, "P12":enum8{"Enabled", "Disabled", "Disabled and Grayed Out"}, "P13":enum8{"Enabled", "Disabled", "Disabled and Grayed Out"}, "P14":enum8{"Enabled", "Disabled", "Disabled and Grayed Out"}, "P15":enum8{"Enabled", "Disabled", "Disabled and Grayed Out"}}, "Cluster Mode CH1":cluster{"#cycles ch1":enum8{"Enabled", "Disabled", "Disabled and Grayed Out"}, "Start ch1":enum8{"Enabled", "Disabled", "Disabled and Grayed Out"}, "Pause ch1":enum8{"Enabled", "Disabled", "Disabled and Grayed Out"}, "Stop ch1":enum8{"Enabled", "Disabled", "Disabled and Grayed Out"}, "Abort ch1":enum8{"Enabled", "Disabled", "Disabled and Grayed Out"}, "Exptime ch1":enum8{"Enabled", "Disabled", "Disabled and Grayed Out"}, "Exp ch1":enum8{"Enabled", "Disabled", "Disabled and Grayed Out"}, "Start ch1 Text":string, "Set Cooler":enum8{"Enabled", "Disabled", "Disabled and Grayed Out"}, "Set Temp":enum8{"Enabled", "Disabled", "Disabled and Grayed Out"}}, "Cluster Mode CH2":cluster{"#cycles ch2":enum8{"Enabled", "Disabled", "Disabled and Grayed Out"}, "Start ch2":enum8{"Enabled", "Disabled", "Disabled and Grayed Out"}, "Pause ch2":enum8{"Enabled", "Disabled", "Disabled and Grayed Out"}, "Stop ch2":enum8{"Enabled", "Disabled", "Disabled and Grayed Out"}, "Abort ch2":enum8{"Enabled", "Disabled", "Disabled and Grayed Out"}, "Exptime ch2":enum8{"Enabled", "Disabled", "Disabled and Grayed Out"}, "Exp ch2":enum8{"Enabled", "Disabled", "Disabled and Grayed Out"}, "Start ch2 Text":string, "Set Cooler":enum8{"Enabled", "Disabled", "Disabled and Grayed Out"}, "Set Temp":enum8{"Enabled", "Disabled", "Disabled and Grayed Out"}}, "Cluster Mode CH3":cluster{"#cycles ch3":enum8{"Enabled", "Disabled", "Disabled and Grayed Out"}, "Start ch3":enum8{"Enabled", "Disabled", "Disabled and Grayed Out"}, "Pause ch3":enum8{"Enabled", "Disabled", "Disabled and Grayed Out"}, "Stop ch3":enum8{"Enabled", "Disabled", "Disabled and Grayed Out"}, "Abort ch3":enum8{"Enabled", "Disabled", "Disabled and Grayed Out"}, "Exptime ch3":enum8{"Enabled", "Disabled", "Disabled and Grayed Out"}, "Exp ch3":enum8{"Enabled", "Disabled", "Disabled and Grayed Out"}, "Start ch3 Text":string, "Set Cooler":enum8{"Enabled", "Disabled", "Disabled and Grayed Out"}, "Set Temp":enum8{"Enabled", "Disabled", "Disabled and Grayed Out"}}, "Cluster Mode CH4":cluster{"#cycles ch4":enum8{"Enabled", "Disabled", "Disabled and Grayed Out"}, "Start ch4":enum8{"Enabled", "Disabled", "Disabled and Grayed Out"}, "Pause ch4":enum8{"Enabled", "Disabled", "Disabled and Grayed Out"}, "Stop ch4":enum8{"Enabled", "Disabled", "Disabled and Grayed Out"}, "Abort ch4":enum8{"Enabled", "Disabled", "Disabled and Grayed Out"}, "Exptime ch4":enum8{"Enabled", "Disabled", "Disabled and Grayed Out"}, "Exp ch4":enum8{"Enabled", "Disabled", "Disabled and Grayed Out"}, "Start ch4 Text":string, "Set Cooler":enum8{"Enabled", "Disabled", "Disabled and Grayed Out"}, "Set Temp":enum8{"Enabled", "Disabled", "Disabled and Grayed Out"}}, "Cluster ExpMode":cluster{"tab4":enum8{"Enabled", "Disabled", "Disabled and Grayed Out"}}, "Cluster AdmCCDsetup":cluster{"param":enum8{"Enabled", "Disabled", "Disabled and Grayed Out"}}}
  T17 = cluster{"broker":string, "version":string, "date":string, "hour":string, "outHumidity":string, "inHumidity":string, "inTemp":string, "outTemp":string, "windSpeed":string, "windDirection":string, "pressure":string, "dewOut":string, "dewIn":string, "leaf":string, "rain":string, "windChill":string}
  T18 = cluster{"WPROT pos":dbl, "WPSEL pos":dbl, "GMIR pos":dbl, "GFOC pos":dbl, "CALW pos":dbl, "ASEL pos":dbl, "mode":bool, "String Status":string, "connection":bool, "operational":bool}
  T19 = cluster{"WPSEL State":i32, "WPROT State":i32, "CALW State":i32, "ASEL State":i32, "GMIR State":i32, "GFOC State":i32}
  T20 = cluster{"WPROT posname":string, "WPSEL posname":string, "CALW posname":string, "ASEL posname":string}
  T21 = cluster{"Current exp":dbl, "Frames done":u32, "LastFileImage":string, "CamStatus":string, "Run state":u32, "connection":bool, "Cooler ON/OFF":i16, "Currently temperature":i16, "Temperature Status":string, "target  temp":i16, "conf runing":bool, "FT":bool, "UsedDisk":u16, "operational":bool}
  T22 = cluster{"Lambda Selector":enum8{"Enabled", "Disabled", "Disabled and Grayed Out"}, "Calibrator Selector":enum8{"Enabled", "Disabled", "Disabled and Grayed Out"}, "Set Waveplate":enum8{"Enabled", "Disabled", "Disabled and Grayed Out"}, "Select Positions":enum8{"Enabled", "Disabled", "Disabled and Grayed Out"}, "P0":enum8{"Enabled", "Disabled", "Disabled and Grayed Out"}, "P1":enum8{"Enabled", "Disabled", "Disabled and Grayed Out"}, "P2":enum8{"Enabled", "Disabled", "Disabled and Grayed Out"}, "P3":enum8{"Enabled", "Disabled", "Disabled and Grayed Out"}, "P4":enum8{"Enabled", "Disabled", "Disabled and Grayed Out"}, "P5":enum8{"Enabled", "Disabled", "Disabled and Grayed Out"}, "P6":enum8{"Enabled", "Disabled", "Disabled and Grayed Out"}, "P7":enum8{"Enabled", "Disabled", "Disabled and Grayed Out"}, "P8":enum8{"Enabled", "Disabled", "Disabled and Grayed Out"}, "P9":enum8{"Enabled", "Disabled", "Disabled and Grayed Out"}, "P10":enum8{"Enabled", "Disabled", "Disabled and Grayed Out"}, "P11":enum8{"Enabled", "Disabled", "Disabled and Grayed Out"}, "P12":enum8{"Enabled", "Disabled", "Disabled and Grayed Out"}, "P13":enum8{"Enabled", "Disabled", "Disabled and Grayed Out"}, "P14":enum8{"Enabled", "Disabled", "Disabled and Grayed Out"}, "P15":enum8{"Enabled", "Disabled", "Disabled and Grayed Out"}}
  T23 = cluster{"#Index Cycles":enum8{"Enabled", "Disabled", "Disabled and Grayed Out"}, "#Cycles":enum8{"Enabled", "Disabled", "Disabled and Grayed Out"}, "SSM":enum8{"Enabled", "Disabled", "Disabled and Grayed Out"}, "Set SM":enum8{"Enabled", "Disabled", "Disabled and Grayed Out"}, "Star SM":enum8{"Enabled", "Disabled", "Disabled and Grayed Out"}, "Pause SM":enum8{"Enabled", "Disabled", "Disabled and Grayed Out"}, "Stop SM":enum8{"Enabled", "Disabled", "Disabled and Grayed Out"}, "Abort SM":enum8{"Enabled", "Disabled", "Disabled and Grayed Out"}, "Start SM Text":string}
  T24 = cluster{"#cycles ch1":enum8{"Enabled", "Disabled", "Disabled and Grayed Out"}, "Start ch1":enum8{"Enabled", "Disabled", "Disabled and Grayed Out"}, "Pause ch1":enum8{"Enabled", "Disabled", "Disabled and Grayed Out"}, "Stop ch1":enum8{"Enabled", "Disabled", "Disabled and Grayed Out"}, "Abort ch1":enum8{"Enabled", "Disabled", "Disabled and Grayed Out"}, "Exptime ch1":enum8{"Enabled", "Disabled", "Disabled and Grayed Out"}, "Exp ch1":enum8{"Enabled", "Disabled", "Disabled and Grayed Out"}, "Start ch1 Text":string, "Set Cooler":enum8{"Enabled", "Disabled", "Disabled and Grayed Out"}, "Set Temp":enum8{"Enabled", "Disabled", "Disabled and Grayed Out"}}
  T25 = cluster{"#cycles ch2":enum8{"Enabled", "Disabled", "Disabled and Grayed Out"}, "Start ch2":enum8{"Enabled", "Disabled", "Disabled and Grayed Out"}, "Pause ch2":enum8{"Enabled", "Disabled", "Disabled and Grayed Out"}, "Stop ch2":enum8{"Enabled", "Disabled", "Disabled and Grayed Out"}, "Abort ch2":enum8{"Enabled", "Disabled", "Disabled and Grayed Out"}, "Exptime ch2":enum8{"Enabled", "Disabled", "Disabled and Grayed Out"}, "Exp ch2":enum8{"Enabled", "Disabled", "Disabled and Grayed Out"}, "Start ch2 Text":string, "Set Cooler":enum8{"Enabled", "Disabled", "Disabled and Grayed Out"}, "Set Temp":enum8{"Enabled", "Disabled", "Disabled and Grayed Out"}}
  T26 = cluster{"#cycles ch3":enum8{"Enabled", "Disabled", "Disabled and Grayed Out"}, "Start ch3":enum8{"Enabled", "Disabled", "Disabled and Grayed Out"}, "Pause ch3":enum8{"Enabled", "Disabled", "Disabled and Grayed Out"}, "Stop ch3":enum8{"Enabled", "Disabled", "Disabled and Grayed Out"}, "Abort ch3":enum8{"Enabled", "Disabled", "Disabled and Grayed Out"}, "Exptime ch3":enum8{"Enabled", "Disabled", "Disabled and Grayed Out"}, "Exp ch3":enum8{"Enabled", "Disabled", "Disabled and Grayed Out"}, "Start ch3 Text":string, "Set Cooler":enum8{"Enabled", "Disabled", "Disabled and Grayed Out"}, "Set Temp":enum8{"Enabled", "Disabled", "Disabled and Grayed Out"}}
  T27 = cluster{"#cycles ch4":enum8{"Enabled", "Disabled", "Disabled and Grayed Out"}, "Start ch4":enum8{"Enabled", "Disabled", "Disabled and Grayed Out"}, "Pause ch4":enum8{"Enabled", "Disabled", "Disabled and Grayed Out"}, "Stop ch4":enum8{"Enabled", "Disabled", "Disabled and Grayed Out"}, "Abort ch4":enum8{"Enabled", "Disabled", "Disabled and Grayed Out"}, "Exptime ch4":enum8{"Enabled", "Disabled", "Disabled and Grayed Out"}, "Exp ch4":enum8{"Enabled", "Disabled", "Disabled and Grayed Out"}, "Start ch4 Text":string, "Set Cooler":enum8{"Enabled", "Disabled", "Disabled and Grayed Out"}, "Set Temp":enum8{"Enabled", "Disabled", "Disabled and Grayed Out"}}
  T28 = cluster{"ACQUISITION_MODE":u8, "TRIGGER_MODE":u8, "READ_MODE":u8, "PREAMP":u8, "READOUT_RATE":u8, "VERTICAL_SHIFT_SPEED":u8, "EM_MODE":u8, "EM_GAIN":u16, "SHUTTER_MODE":u8, "SHUTTER_TTL":u8, "SHUTTER_OPENNING_TIME":u16, "SHUTTER_CLOSING_TIME":u16, "VBIN":u16, "HBIN":u16, "INITIAL_LINE":u16, "INITIAL_COLUMN":u16, "FINAL_LINE":u16, "FINAL_COLUMN":u16, "FRAME_TRANSFER":bool, "VERTICAL_CLOCK_VOLTAGE":u8, "AD_CHANNEL":u32}
  T29 = cluster{"SZM":enum16{"LARGE: FoV=5.6' / Pix=0.3\"", "LARGE: FoV=5.6' / Pix=0.7\"", "MEDIUM: FoV=2.8'/ Pix=0.3\"", "MEDIUM: FoV=2.8' / Pix=0.7\"", "SMALL FoV=1.4' / Pix=0.3\"", "SMALL: FoV=1.4' / Pix=0.7\""}, "AQM":enum16{"SLOW BRIGHT: Conventional; 0.1 MHz; Gain 1", "SLOW FAINT: Conventional; 0.1 MHz; Gain 2", "NORMAL BRIGHT: Conventional; 1 MHz; Gain 1", "NORMAL FAINT: Conventional; 1 MHz; Gain 2", "FAST: EM; 10 MHz", "FAST+: EM; 20 MHz", "SUPERFAST: EM; 30 MHz"}, "FTM":enum16{"OFF", "ON"}, "EM gain":u16}
  T30 = cluster{"ACQUISITION_MODE":u8, "TRIGGER_MODE":u8, "READ_MODE":u8, "PREAMP":u8, "READOUT_RATE":u8, "VERTICAL_SHIFT_SPEED":u8, "EM_MODE":u8, "EM_GAIN":u16, "SHUTTER_MODE":u8, "SHUTTER_TTL":u8, "SHUTTER_OPENING_TIME":u16, "SHUTTER_CLOSING_TIME":u16, "VBIN":u16, "HBIN":u16, "INITIAL_LINE":u16, "INITIAL_COLUMN":u16, "FINAL_LINE":u16, "FINAL_COLUMN":u16, "FRAME_TRANSFER":bool, "VERTICAL_CLOCK_VOLTAGE":u8, "AD_CHANNEL":u32}
  T31 = cluster{"Image Initial Line":dbl, "Image Initial Column":dbl, "Image Final Line":dbl, "Image FInal Column":dbl, "Vertical Binning":dbl, "Horizontal Binning":dbl, "Pre-amplification Gain":u8, "CCD EM Gain":u8, "Readout Rate":u8, "Shutter Openning Time":i32, "Shutter Closing Time":i32, "Vertical Shift Speed":u8, "Read Mode":u8, "Vertical Clock Voltage":u8, "A/D  Channel":u32, "Image Initial Line 2":dbl, "Image Initial Column 2":dbl, "Image Final Line 2":dbl, "Image FInal Column 2":dbl, "Vertical Binning 2":dbl, "Horizontal Binning 2":dbl, "Pre-amplification Gain 2":u8, "CCD EM Gain 2":u16, "Readout Rate 2":u8, "Shutter Openning Time 2":i32, "Shutter Closing Time 2":i32, "Vertical Shift Speed 2":u8, "Read Mode 2":u8, "Vertical Clock Voltage 2":u8, "A/D Channel 2":u32, "Image Initial Line 3":dbl, "Image Initial Column 3":dbl, "Image Final Line 3":dbl, "Image FInal Column 3":dbl, "Vertical Binning 3":dbl, "Horizontal Binning 3":dbl, "Pre-amplification Gain 3":u8, "CCD EM Gain 3":u16, "Readout Rate 3":u8, "Shutter Openning Time 3":i32, "Shutter Closing Time 3":i32, "Vertical Shift Speed 3":u8, "Read Mode 3":u8, "Vertical Clock Voltage 3":u8, "A/D Channel 3":u32, "Image Initial Line 4":dbl, "Image Initial Column 4":dbl, "Image Final Line 4":dbl, "Image FInal Column 4":dbl, "Vertical Binning 4":dbl, "Horizontal Binning 4":dbl, "Pre-amplification Gain 4":u8, "CCD EM Gain 4":u16, "Readout Rate 4":u8, "Shutter Openning Time 4":i32, "Shutter Closing Time 4":i32, "Vertical Shift Speed 4":u8, "Read Mode 4":u8, "Vertical Clock Voltage 4":u8, "A/D Channel 4":u32, "CCD EM Mode 2":u8, "CCD EM Mode 3":u8, "CCD EM Mode 4":u8, "CCD EM Mode":u16, "Shutter Mode":u16, "Shutter Mode 2":u16, "Shutter Mode 4":u16, "Shutter Mode 3":u16, "Shutter TTL":u16, "Shutter TTL 2":u16, "Shutter TTL 3":u16, "Shutter TTL 4":u16, "Frame Transfer":bool, "Frame Transfer 2":bool, "Frame Transfer 3":bool, "Frame Transfer 4":bool, "Trigger Mode":u16, "Trigger Mode 2":u16, "Trigger Mode 3":u16, "Trigger Mode 4":u16, "Acquisition Mode":u8, "Acquisition Mode 2":u8, "Acquisition Mode 3":u8, "Acquisition Mode 4":u8}
